vi "Test Make and Run Suite from Test Case Inherits Tests.vi"(8 "error in (no error)":errorcluster, 11 "Test Case In":refnum<class "Inheritance Test.lvclass">) -> (0 "error out":errorcluster, 3 "Test Case Out":refnum<class "Inheritance Test.lvclass">)   [LabVIEW 2020, in "Inheritance Test.lvclass"]
uses:
  Inheritance Test.lvclass
  C:/Program Files (x86)/National Instruments/LabVIEW 2020/vi.lib/Astemes/LUnit/Test Case.lvclass
  Test Doubles/Test Case Test Double/Test Case Test Double Child.lvclass
  <vilib>/Astemes/LUnit/Test Case.lvclass/Test Case.ctl
  c58b3855-ebe9-4a85-9df9-c2f1dfef19ff.vi
  <vilib>/Astemes/LUnit/Append Pass Result.vi
  <vilib>/Astemes/LUnit/Append Fail Result.vi
  <vilib>/Astemes/LUnit/Describe Comparison.vi
  <vilib>/Astemes/LUnit/Compare Variants.vi
  <vilib>/Astemes/LUnit/Run In UI.vi
  <vilib>/Utility/error.llb/Clear Errors.vi
  <vilib>/Astemes/LUnit/Describe Variant.vi
  <vilib>/Astemes/LUnit/Test Suite.lvclass
  Inheritance Test.lvclass/Inheritance Test.ctl
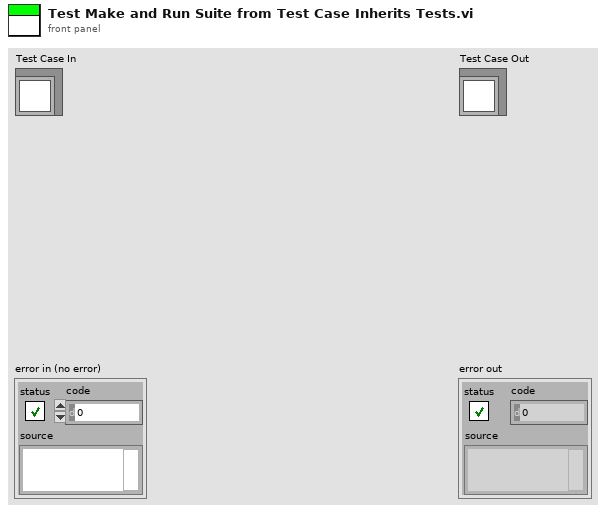
[diagram p1: front panel]
types:
  T1 = enum16{"Test Case", "Test Suite", "Test Run", "Pass", "Fail", "Skip", "Pass if", "Fail if", "Pass if Error", "Fail if Error", "Pass if Equal", "Fail if Equal"}
  T2 = cluster{"Name":string, "Message":string, "Description":string, "Status":enum16{"", "Passed", "Failed", "Error", "Skipped", "Setup Error", "Broken", "Teardown Error"}, "Result Type":enum16{"Test Case", "Test Suite", "Test Run", "Pass", "Fail", "Skip", "Pass if", "Fail if", "Pass if Error", "Fail if Error", "Pass if Equal", "Fail if Equal"}, "Execution Time":dbl}[]
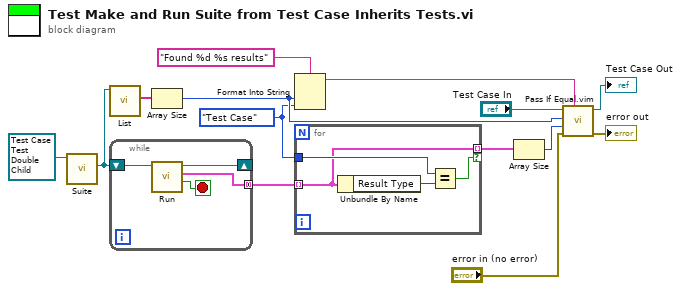
[diagram p0: block diagram]
diagram:
  w2 = T1."Test Case" ("x")
  n1 = call-dynamic "Suite.vi"("LUnit Test Case in"=refnum<class "Test Case Test Double Child.lvclass"> refnum ("Test Case Test Double Child.lvclass")) -> ("LUnit Test Suite Out"=w8:refnum<class "Test Suite.lvclass">)  [unwired: 8 in, 2 out]
  n2 = call <vilib>:"List.vi"("LUnit Test Suite In"=w8) -> ("List of Runnables"=w7:string[])  [unwired: 9 in, 1 out]
  n3 = while {
    tunnel: [w18] -> w9 mode=concatenating
    shift-right: [w15] -> _
    shift-left: w8 -> [w17]
    stop <- w16 stop-if-true
    n4 = call-dynamic "Run.vi"("LUnit Test Suite In"=w17) -> ("Done?"=w16:bool, "Results"=w18:T2, "LUnit Test Suite In 2"=w15:refnum<class "Test Suite.lvclass">)  [unwired: 7 in, 1 out]
  }
  n5 = Array Size(array=w7) -> (size(s)=w6:i32)
  n6 = Format Into String(format string="Found %d %s results", w6, w2) -> (resulting string=w1:string)  [unwired: 2 in, 1 out]
  n7 = for {
    tunnel: w9 -> [w20] mode=indexing
    tunnel: w2 -> [w21]
    tunnel: [w20] -> w5 mode=indexing if=w19
    n8 = Unbundle By Name(w20) -> ("Result Type"=w22:T1)
    n9 = Equal?(x=w21, y=w22) -> (x = y?=w19:bool)
  }
  n10 = Array Size(array=w5) -> (size(s)=w4:i32)
  n11 = call "Pass If Equal.vim"("Description"=w1, "error in (no error)"="error in (no error)", "Actual"=w4, "Expected"=w6, "LUnit Test Case In"="Test Case In") -> ("error out"=→"error out":errorcluster, "LUnit Test Case Out"=→"Test Case Out":refnum<class "Inheritance Test.lvclass">)  [unwired: 5 in]
